vi "Abort Multipart Upload.vi"(8 "error in (no error)":errorcluster, 11 "Multipart Upload":refnum<class "Multipart Upload.lvclass">) -> (0 "error out":errorcluster, 3 "Bucket":refnum<class "Bucket.lvclass">)   [LabVIEW 2015, in "NI_AWS_S3.lvlib" / "Multipart Upload.lvclass"]
uses:
  Multipart Upload.lvclass
  Bucket/Bucket.lvclass
  Core/HTTP Request/Name Value Pair.ctl
  Core/HTTP Request/Request Options.ctl
  Core/HTTP Request/Region handling.ctl
  Core/HTTP Request/URL formatting.ctl
  Multipart Upload.lvclass/Multipart Upload.ctl
  Bucket/Bucket.lvclass/Bucket.ctl
  Read Bucket.vi
  Read Upload ID.vi
  Read Object Key.vi
  Bucket/Read Name.vi
  Core/HTTP Request/HTTP Request.lvclass
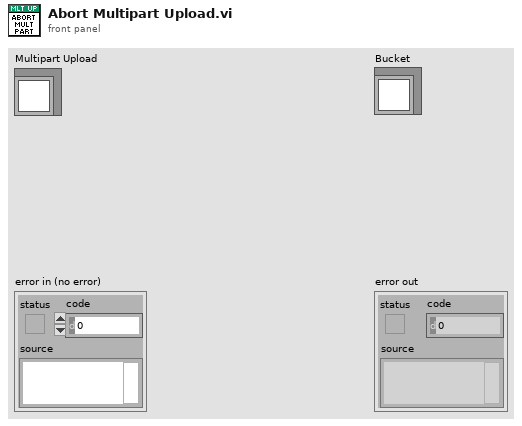
[diagram p1: front panel]
types:
  T1 = typedef "NI_AWS_Core.lvlib/HTTP Request.lvclass/Region handling.ctl" = enum16{"use region everywhere", "use region (authentication only)", "use region (URL only)", "ignore region everwhere"}
  T2 = typedef "NI_AWS_Core.lvlib/HTTP Request.lvclass/Request Options.ctl" = cluster{"request headers":T3[], "request parameters":T3[], "request body":string, "region handling":T1, "URL formatting":T4}
  T3 = typedef "NI_AWS_Core.lvlib/HTTP Request.lvclass/Name Value Pair.ctl" = cluster{"name":string, "value":string}
  T4 = typedef "NI_AWS_Core.lvlib/HTTP Request.lvclass/URL formatting.ctl" = enum16{"region-", "region."}
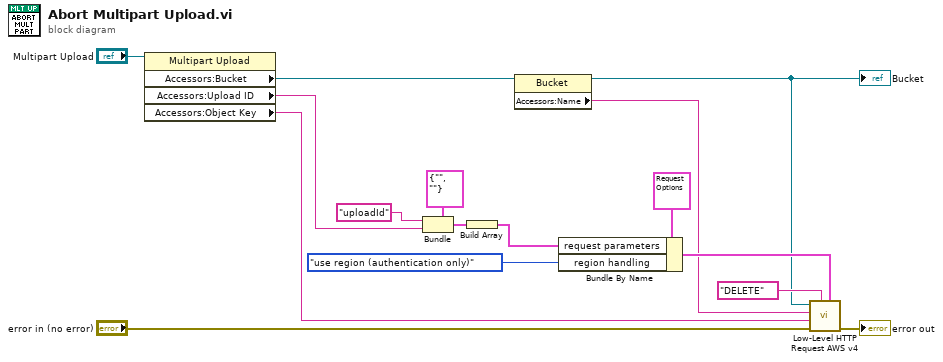
[diagram p0: block diagram]
diagram:
  n1 = property class="Multipart Upload"(reference="Multipart Upload") -> ("Accessors:Bucket"=w7:refnum<class "Bucket.lvclass">, "Accessors:Upload ID"=w1:string, "Accessors:Object Key"=w4:string)  [unwired: 1 in, 2 out]
  n2 = Bundle(cluster=T3 {"name"="", "value"=""} ("Name Value Pair"), "name"="uploadId" ("format string"), "value"=w1) -> (w15:T3)
  n3 = Build Array(w15) -> (w2:T3[])
  n4 = property class="Bucket"(reference=w7) -> (reference out=w6:refnum<class "Bucket.lvclass">, "Accessors:Name"=w5:string)  [unwired: 1 in, 1 out]
  "Bucket" <- w6
  n5 = Bundle By Name(cluster=T2 {"request headers"=[], "request parameters"=[], "request body"="", "region handling"=enum."use region everywhere", "URL formatting"=enum."region."} ("Request Options"), "request parameters"=w2, "region handling"=Region_handling."use region (authentication only)") -> (w11:T2)
  n6 = call "Low-Level HTTP Request AWS v4.vi"("Request Options"=w11, "HTTP-Verb"="DELETE", "error in (no error)"="error in (no error)", "URL Suffix"=w4, "URL Prefix"=w5, "AWS Core in"=w6) -> ("error out"=→"error out":errorcluster)  [unwired: 2 in, 3 out]
